vi "limelightLoop.vi"   [LabVIEW 2018]
uses:
  <vilib>/Platform/TimedLoop/XDataNode/timing_clust.ctl
  <vilib>/Platform/TimedLoop/XDataNode/nitl_modes.ctl
  <vilib>/Platform/TimedLoop/XDataNode/wakeup.ctl
  LimelightModeEnum.ctl
  <userlib>/836-Library/System/TDMS_V2/Support/TDMS_DevRef.ctl
  <userlib>/836-Library/System/TDMS_V2/Support/Logging_Settings.ctl
  <userlib>/836-Library/System/TDMS_V2/Support/Group_FIFO_Config.ctl
  <userlib>/836-Library/System/TDMS_V2/Support/Channel_FIFO_Config.ctl
  LimelightNTStream.ctl
  LimelightNTCamMode.ctl
  LimelightNTLEDMode.ctl
  <vilib>/Rock Robotics/Network Tables/NT Read Number.vi
  <vilib>/Rock Robotics/Network Tables/NT Write Number.vi
  <vilib>/platform/TimedLoop/XDataNode/XDataNode.xnode
  <vilib>/Platform/TimedLoop/XDataNode/XDNodeRunTimeDep.lvlib
types:
  T1 = typedef "XDNodeRunTimeDep.lvlib/timing_clust.ctl" = cluster{"Expected End [f-1]":u64, "Actual End [f-1]":u64, "Finished Late? [f-1]":bool, "Expected End [i-1]":u64, "Actual End [i-1]":u64, "Finished Late? [i-1]":bool, "Expected Start [i]":u64, "Actual Start [i]":u64, "Expected Start [f]":u64, "Actual Start [f]":u64, "Source Name":string, "Structure Name":string, "Period":i64, "Deadline":i64, "Offset":i64, "Start":i64, "Priority":i32, "Timeout":i32, "Mode":T2, "Wakeup Reason":T3, "Error":errorcluster, "Source Type":string, "Secondary Source Type":string, "Global End Time":u64, "Global Start Time":u64, "Frame Duration":u64, "Iteration Duration":u64, "Assigned CPU":i32, "I/O Scan Engine Mode":u32}
  T2 = typedef "XDNodeRunTimeDep.lvlib/nitl_modes.ctl" = enum32{"No Change", "Process missed periods, maintain original phase", "Discard missed periods, maintain original phase", "Process missed periods, ignore original phase", "Discard missed periods, ignore original phase"}
  T3 = typedef "XDNodeRunTimeDep.lvlib/wakeup.ctl" = enum32{"Normal", "Aborted", "Asynchronous wakeup", "Timing source error", "Timed loop error", "Timeout"}
  T4 = typedef "LimelightModeEnum.ctl" = enum16{"SA - Front", "SA - Rear", "SA - Side by Side", "Vision Processing"}
  T5 = typedef "LimelightNTLEDMode.ctl" = enum16{"Pipeline Mode", "Force Off", "Blink", "Force On"}
  T6 = typedef "LimelightNTStream.ctl" = enum16{"Standard - Side by Side", "PiP Main", "PiP Secondary"}
  T7 = typedef "LimelightNTCamMode.ctl" = enum16{"Vision Processing", "Driver Camera"}
  T8 = typedef "TDMS_DevRef.ctl" = cluster{"Name":string, "File Ref":refnum<k34>, "Start Time":timestamp, "Logging Settings":T9, "Group FIFO Config":T10[], "Data To Write":refnum<data-value>, "semaphore":T12, "Ref Time Reset":refnum<k4>}
  T9 = typedef "Logging_Settings.ctl" = cluster{"Data Grab Period":dbl, "File Write Period":dbl, "Max Stored Size":dbl, "Burst Size":dbl}
  T10 = typedef "Group_FIFO_Config.ctl" = cluster{"Group":string, "Channels":T11[], "Channel Names":string[]}
  T11 = typedef "Channel_FIFO_Config.ctl" = cluster{"Channel":string, "FIFO":refnum<k33>}
  T12 = typedef "Semaphore RefNum" = refnum<k1>
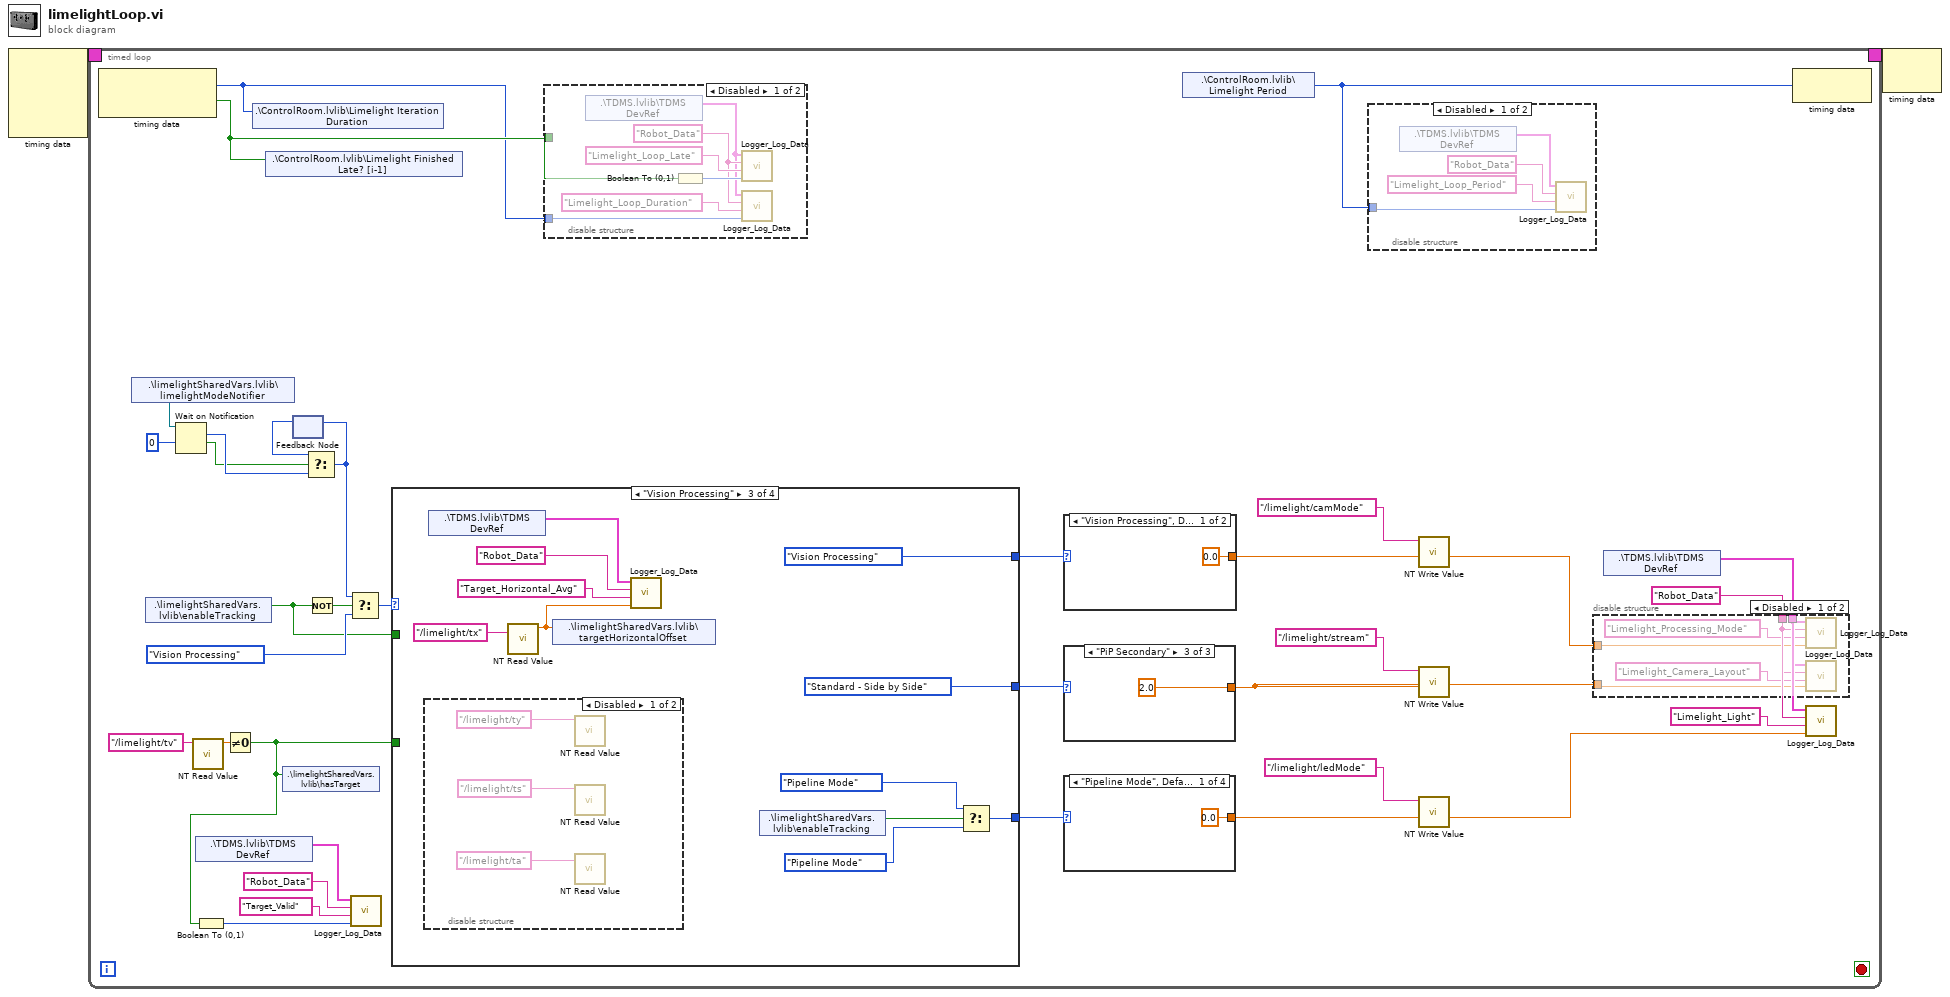
[diagram p0: block diagram]
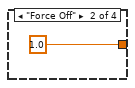
[diagram p3: hidden frame]
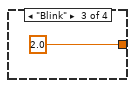
[diagram p4: hidden frame]
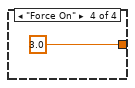
[diagram p5: hidden frame]
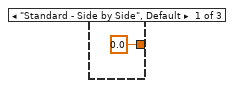
[diagram p6: hidden frame]
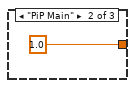
[diagram p7: hidden frame]
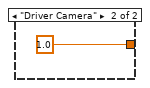
[diagram p8: hidden frame]
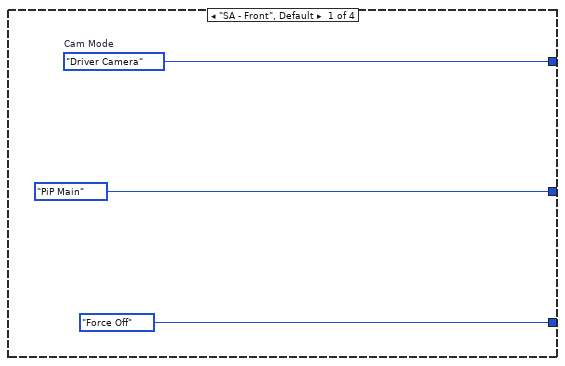
[diagram p9: hidden frame]
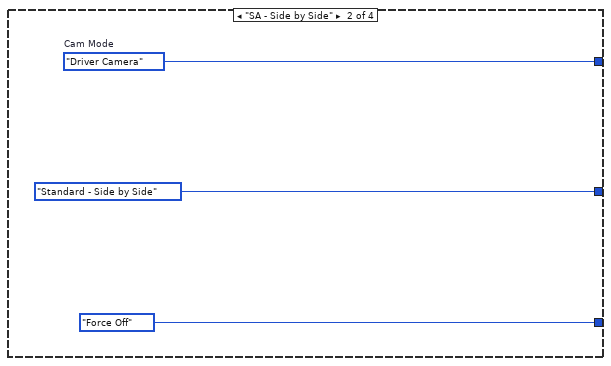
[diagram p10: hidden frame]
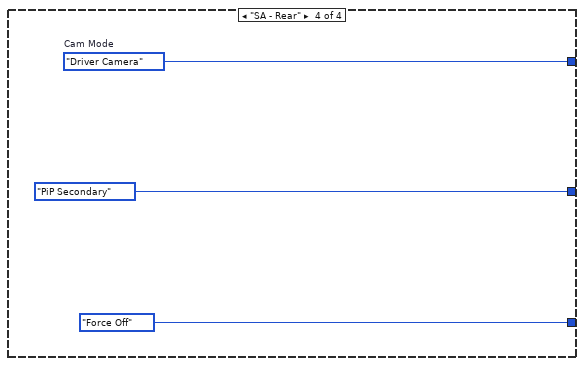
[diagram p12: hidden frame]
diagram:
  n1 = node-c288() -> (w2:T1)  [unwired: 4 in]
  n2 = timed-loop {
    timing: w2 -> [_]
    timing-out: [_] -> w1
    stop <- _ stop-if-true
    w10 = "Robot_Data" ("Group")
    n3 = node-c288() -> (w26:i64, w27:bool)  [unwired: 1 in]
    n4 = shared-variable ".\\limelightSharedVars.lvlib\\limelightModeNotifier"() -> (w33:refnum<notifier>)  [unwired: 1 in, 1 out]
    n5 = shared-variable ".\\limelightSharedVars.lvlib\\enableTracking"() -> (w13:bool)  [unwired: 1 in, 1 out]
    n6 = Wait on Notification(notifier=w33, timeout in ms (-1)=0) -> (notification=w31:T4, timed out?=w30:bool)  [unwired: 2 in, 2 out]
    n7 = call-poly <vilib>:"NT Read Value.vi"("Name"="/limelight/tv") -> ("Numeric"=w9:dbl)  [unwired: 9 in, 1 out]
    n8 = shared-variable ".\\TDMS.lvlib\\TDMS DevRef"() -> (w6:T8)  [unwired: 1 in, 1 out]
    n9 = Not Equal To 0?(x=w9) -> (x != 0?=w3:bool)
    n10 = Boolean To (0,1)(Boolean=w3) -> (0, 1=w5:i16)
    n11 = shared-variable ".\\ControlRoom.lvlib\\Limelight Iteration Duration"(w26) -> ()  [unwired: 1 in, 1 out]
    n12 = shared-variable ".\\ControlRoom.lvlib\\Limelight Finished Late? [i-1]"(w27) -> ()  [unwired: 1 in, 1 out]
    n13 = shared-variable ".\\limelightSharedVars.lvlib\\hasTarget"(w3) -> ()  [unwired: 1 in, 1 out]
    n14 = feedback #1() -> (w32:T4)  [unwired: 1 in]
    n15 = Select(t=w32, s=w30, f=w31) -> (s? t:f=w24:T4)
    n16 = feedback-in #1(w24) -> ()
    n17 = Not(x=w13) -> (.not. x?=w23:bool)
    n18 = Select(t=w24, s=w23, f=LimelightModeEnum."Vision Processing") -> (s? t:f=w29:T4)
    n19 = call <userlib>:"Logger_Log_Data.vi"("Data"=w5, "Channel"="Target_Valid", "Group"="Robot_Data", "TDMS DevRef"=w6) -> ()  [unwired: 7 in, 1 out]
    n20 = case shown="\"Vision Processing\"" w29 {
      tunnel: [w51 w54 LimelightNTCamMode."Vision Processing" ("Cam Mode") w71] -> w19
      tunnel: [LimelightNTStream."PiP Main" LimelightNTStream."Standard - Side by Side" LimelightNTStream."Standard - Side by Side" LimelightNTStream."PiP Secondary"] -> w17
      tunnel: [LimelightNTLEDMode."Force Off" ("LED Mode") LimelightNTLEDMode."Force Off" ("LED Mode") w64 LimelightNTLEDMode."Force Off" ("LED Mode")] -> w18
      tunnel: w13 -> [_ _ _ _]
      tunnel: w3 -> [_ _ _ _]
      frame "SA - Front", Default {
        w51 = LimelightNTCamMode."Driver Camera"  # Cam Mode
      }
      frame "SA - Side by Side" {
        w54 = LimelightNTCamMode."Driver Camera"  # Cam Mode
      }
      frame "Vision Processing" {
        n21 = disable-structure shown="Disabled" {
          frame Disabled {
            n22 = call-poly <vilib>:"NT Read Value.vi"("Name"="/limelight/ty") -> ()  [unwired: 9 in, 2 out]
            n23 = call-poly <vilib>:"NT Read Value.vi"("Name"="/limelight/ts") -> ()  [unwired: 9 in, 2 out]
            n24 = call-poly <vilib>:"NT Read Value.vi"("Name"="/limelight/ta") -> ()  [unwired: 9 in, 2 out]
          }
          frame Enabled {
          }
        }
        n25 = shared-variable ".\\TDMS.lvlib\\TDMS DevRef"() -> (w58:T8)  [unwired: 1 in, 1 out]
        n26 = call-poly <vilib>:"NT Read Value.vi"("Name"="/limelight/tx") -> ("Numeric"=w56:dbl)  [unwired: 9 in, 1 out]
        n27 = shared-variable ".\\limelightSharedVars.lvlib\\targetHorizontalOffset"(w56) -> ()  [unwired: 1 in, 1 out]
        n28 = call <userlib>:"Logger_Log_Data.vi"("Data"=w56, "Channel"="Target_Horizontal_Avg", "Group"="Robot_Data", "TDMS DevRef"=w58) -> ()  [unwired: 7 in, 1 out]
        n29 = shared-variable ".\\limelightSharedVars.lvlib\\enableTracking"() -> (w63:bool)  [unwired: 1 in, 1 out]
        n30 = Select(t=LimelightNTLEDMode."Pipeline Mode" ("LED Mode"), s=w63, f=LimelightNTLEDMode."Pipeline Mode") -> (s? t:f=w64:T5)
      }
      frame "SA - Rear" {
        w71 = LimelightNTCamMode."Driver Camera"  # Cam Mode
      }
    }
    n31 = disable-structure shown="Disabled" {
      disable-tunnel: w27 -> [w83 _]
      disable-tunnel: w26 -> [w82 _]
      frame Disabled {
        w78 = "Robot_Data" ("Group")
        n32 = shared-variable ".\\TDMS.lvlib\\TDMS DevRef"() -> (w77:T8)  [unwired: 1 in, 1 out]
        n33 = Boolean To (0,1)(Boolean=w83) -> (0, 1=w80:i16)
        n34 = call <userlib>:"Logger_Log_Data.vi"("Data"=w80, "Channel"="Limelight_Loop_Late", "Group"=w78, "TDMS DevRef"=w77) -> ()  [unwired: 7 in, 1 out]
        n35 = call <userlib>:"Logger_Log_Data.vi"("Data"=w82, "Channel"="Limelight_Loop_Duration", "Group"=w78, "TDMS DevRef"=w77) -> ()  [unwired: 7 in, 1 out]
      }
      frame Enabled {
      }
    }
    n36 = case shown="\"Vision Processing\", Default" w19 {
      tunnel: [0.0 1.0] -> w15
      frame "Vision Processing", Default {
      }
      frame "Driver Camera" {
      }
    }
    n37 = case shown="\"PiP Secondary\"" w17 {
      tunnel: [0.0 1.0 2.0] -> w16
      frame "Standard - Side by Side", Default {
      }
      frame "PiP Main" {
      }
      frame "PiP Secondary" {
      }
    }
    n38 = case shown="\"Pipeline Mode\", Default" w18 {
      tunnel: [0.0 1.0 2.0 3.0] -> w14
      frame "Pipeline Mode", Default {
      }
      frame "Force Off" {
      }
      frame "Blink" {
      }
      frame "Force On" {
      }
    }
    n39 = shared-variable ".\\ControlRoom.lvlib\\Limelight Period"() -> (w25:i64)  [unwired: 1 in, 1 out]
    n40 = disable-structure shown="Disabled" {
      disable-tunnel: w25 -> [w76 _]
      frame Disabled {
        n41 = shared-variable ".\\TDMS.lvlib\\TDMS DevRef"() -> (w74:T8)  [unwired: 1 in, 1 out]
        n42 = call <userlib>:"Logger_Log_Data.vi"("Data"=w76, "Channel"="Limelight_Loop_Period", "Group"="Robot_Data", "TDMS DevRef"=w74) -> ()  [unwired: 7 in, 1 out]
      }
      frame Enabled {
      }
    }
    n43 = call-poly <vilib>:"NT Write Value.vi"("Numeric"=w15, "Name"="/limelight/camMode") -> ()  [unwired: 9 in, 1 out]
    n44 = call-poly <vilib>:"NT Write Value.vi"("Numeric"=w16, "Name"="/limelight/stream") -> ()  [unwired: 9 in, 1 out]
    n45 = call-poly <vilib>:"NT Write Value.vi"("Numeric"=w14, "Name"="/limelight/ledMode") -> ()  [unwired: 9 in, 1 out]
    n46 = shared-variable ".\\TDMS.lvlib\\TDMS DevRef"() -> (w11:T8)  [unwired: 1 in, 1 out]
    n47 = disable-structure shown="Disabled" {
      disable-tunnel: w16 -> [w40 _]
      disable-tunnel: w15 -> [w39 _]
      disable-tunnel: w11 -> [w36 _]
      disable-tunnel: w10 -> [w35 _]
      frame Disabled {
        n48 = call <userlib>:"Logger_Log_Data.vi"("Data"=w39, "Channel"="Limelight_Processing_Mode", "Group"=w35, "TDMS DevRef"=w36) -> ()  [unwired: 7 in, 1 out]
        n49 = call <userlib>:"Logger_Log_Data.vi"("Data"=w40, "Channel"="Limelight_Camera_Layout", "Group"=w35, "TDMS DevRef"=w36) -> ()  [unwired: 7 in, 1 out]
      }
      frame Enabled {
      }
    }
    n50 = node-c288(w25) -> ()  [unwired: 1 out]
    n51 = call <userlib>:"Logger_Log_Data.vi"("Data"=w14, "Channel"="Limelight_Light", "Group"=w10, "TDMS DevRef"=w11) -> ()  [unwired: 7 in, 1 out]
  }
  n52 = node-c288(w1) -> ()  [unwired: 1 out]
